vi "Add PID Controller.vi"(8 "error in (no error)":errorcluster, 11 "Node Ptr":u64 format="%.0x") -> (0 "error out":errorcluster)   [LabVIEW 2013, in "Control Addon System Explorer.lvlib"]
uses:
  Control Addon System Explorer.lvlib
  <vilib>/NI Veristand/Custom Device API/Custom Device Channel.ctl
  <vilib>/NI Veristand/Custom Device API/Custom Device Channel Type.ctl
  Shared/Constants.vi
  <vilib>/NI Veristand/Custom Device API/Custom Device API.lvlib
  Shared/Control Addon Shared.lvlib
panel:
  in  "Tag":string
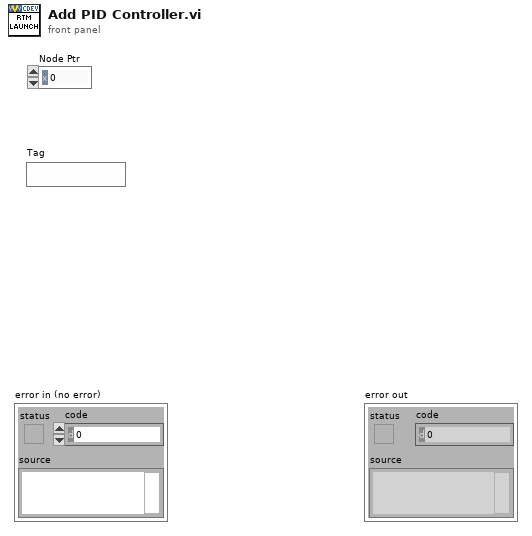
[diagram p1: front panel]
types:
  T1 = typedef "Custom Device API.lvlib/Custom Device Channel.ctl" = cluster{"Type":T2, "Units":string, "Default Value":dbl, "Faultable":bool, "Scalable":bool}
  T2 = typedef "Custom Device API.lvlib/Custom Device Channel Type.ctl" = enum16{"Input", "Output"}
  T3 = typedef "Custom Device API.lvlib/Custom Device Item Ref.ctl" = u64
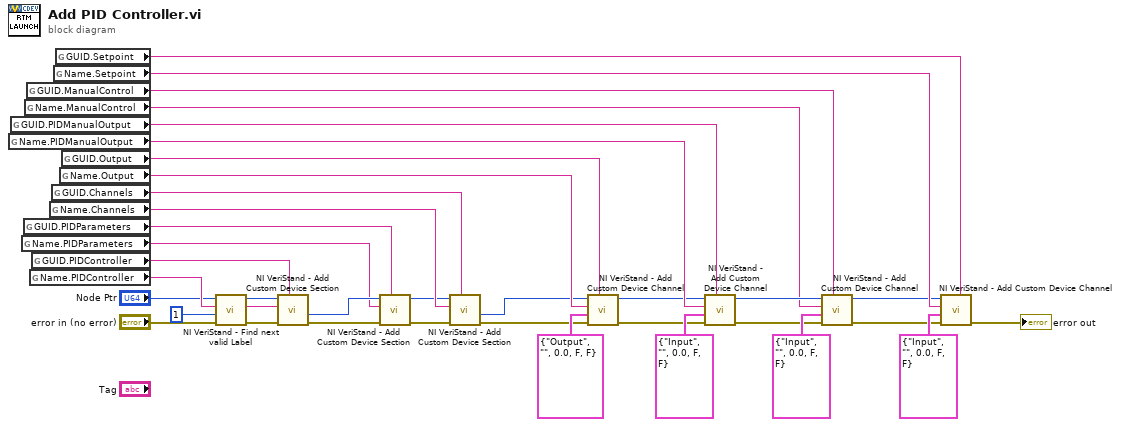
[diagram p0: block diagram]
diagram:
  n1 = global read "Constants.vi" "Name.PIDManualOutput"() -> (w11:string)
  n2 = global read "Constants.vi" "GUID.PIDManualOutput"() -> (w7:string)
  n3 = global read "Constants.vi" "Name.PIDParameters"() -> (w32:string)
  n4 = global read "Constants.vi" "GUID.PIDParameters"() -> (w31:string)
  n5 = global read "Constants.vi" "Name.ManualControl"() -> (w10:string)
  n6 = global read "Constants.vi" "GUID.ManualControl"() -> (w9:string)
  n7 = global read "Constants.vi" "Name.PIDController"() -> (w28:string)
  n8 = global read "Constants.vi" "GUID.PIDController"() -> (w35:string)
  n9 = global read "Constants.vi" "Name.Channels"() -> (w19:string)
  n10 = global read "Constants.vi" "GUID.Channels"() -> (w20:string)
  n11 = global read "Constants.vi" "Name.Setpoint"() -> (w29:string)
  n12 = global read "Constants.vi" "GUID.Setpoint"() -> (w6:string)
  n13 = global read "Constants.vi" "Name.Output"() -> (w30:string)
  n14 = global read "Constants.vi" "GUID.Output"() -> (w8:string)
  n15 = call <vilib>:"NI VeriStand - Find next valid Label.vi"("error in (no error)"="error in (no error)", "Start Value (1)"=1, "Label"=w28, "Item Ref in"="Node Ptr") -> ("error out"=w23:errorcluster, "Label out"=w27:string, "Item Ref out"=w25:T3)  [unwired: 3 in, 2 out]
  n16 = call <vilib>:"NI VeriStand - Add Custom Device Section.vi"("GUID (Default Section)"=w35, "error in (no error)"=w23, "Section Name"=w27, "Parent Ref in"=w25) -> ("error out"=w37:errorcluster, "Section Ptr"=w36:T3)  [unwired: 4 in, 2 out]
  n17 = call <vilib>:"NI VeriStand - Add Custom Device Section.vi"("GUID (Default Section)"=w31, "error in (no error)"=w37, "Section Name"=w32, "Parent Ref in"=w36) -> ("error out"=w16:errorcluster, "Parent Ref out"=w17:T3)  [unwired: 4 in, 2 out]
  n18 = call <vilib>:"NI VeriStand - Add Custom Device Section.vi"("GUID (Default Section)"=w20, "error in (no error)"=w16, "Section Name"=w19, "Parent Ref in"=w17) -> ("error out"=w22:errorcluster, "Section Ptr"=w21:T3)  [unwired: 4 in, 2 out]
  n19 = call <vilib>:"NI VeriStand - Add Custom Device Channel.vi"("GUID (Default Channel)"=w8, "error in (no error)"=w22, "Channel"=T1 {"Type"=enum."Output", "Units"="", "Default Value"=0.0, "Faultable"=FALSE, "Scalable"=FALSE}, "Channel Name"=w30, "Parent Ref in"=w21) -> ("error out"=w4:errorcluster, "Parent Ref out"=w5:T3)  [unwired: 3 in, 2 out]
  n20 = call <vilib>:"NI VeriStand - Add Custom Device Channel.vi"("GUID (Default Channel)"=w7, "error in (no error)"=w4, "Channel"=T1 {"Type"=enum."Input", "Units"="", "Default Value"=0.0, "Faultable"=FALSE, "Scalable"=FALSE}, "Channel Name"=w11, "Parent Ref in"=w5) -> ("error out"=w13:errorcluster, "Parent Ref out"=w12:T3)  [unwired: 3 in, 2 out]
  n21 = call <vilib>:"NI VeriStand - Add Custom Device Channel.vi"("GUID (Default Channel)"=w9, "error in (no error)"=w13, "Channel"=T1 {"Type"=enum."Input", "Units"="", "Default Value"=0.0, "Faultable"=FALSE, "Scalable"=FALSE}, "Channel Name"=w10, "Parent Ref in"=w12) -> ("error out"=w2:errorcluster, "Parent Ref out"=w1:T3)  [unwired: 3 in, 2 out]
  n22 = call <vilib>:"NI VeriStand - Add Custom Device Channel.vi"("GUID (Default Channel)"=w6, "error in (no error)"=w2, "Channel"=T1 {"Type"=enum."Input", "Units"="", "Default Value"=0.0, "Faultable"=FALSE, "Scalable"=FALSE}, "Channel Name"=w29, "Parent Ref in"=w1) -> ("error out"=→"error out":errorcluster)  [unwired: 3 in, 3 out]
